vi "Unicode Read Text File Example.vi"() -> ()   [LabVIEW 2020]
doc: "This example demonstrates reading and displaying unicode text from a file."
uses:
  Unicode/Controls/String Encoding.ctl
  Types/UTF-8 Path/UTF-8 Path.lvclass/UTF-8 Path.ctl
  Types/UTF-8 String/UTF-8 String.lvclass/UTF-8 String.ctl
  Types/UTF-8 String/UTF-8 String.lvclass
  Types/UTF-8 Path/UTF-8 Path.lvclass
  815672e0-49fd-43dc-9208-6db65f057bb6.vi
  b6c8d447-eb94-4308-a095-128f48e3c673.vi
  56f3dc87-de23-4d90-98a5-7b236af5e5d4.vi
  45627e68-18eb-4edc-9747-f3175908f235.vi
  Dialog & User Interface/Polymorphic VIs/Write Control Text/Write String Value (UTF-8 String).vi
  Private/Conversion/Text as Encoded Path.vi
  Private/Conversion/Polymorphic VIs/Text as Encoded Path (LabVIEW Path).vi
  Types/UTF-8 Path/Write Encoded UTF-8 Path.vi
  Private/Conversion/Path as Encoded Path.vi
  Private/Conversion/Polymorphic VIs/Path as Encoded Path (LabVIEW Path).vi
  Private/Conversion/String as Encoded String.vi
  Private/Conversion/Polymorphic VIs/String as Encoded String (LabVIEW String).vi
  Private/Conversion/Text as Encoded String.vi
  Private/Conversion/Polymorphic VIs/Text as Encoded String (UTF-8 Path).vi
  Private/Library/gu_open_file_dialog.vi
  Private/Library/gu_select_folder_dialog.vi
  Private/Conversion/Path as UTF-8 Path.vi
  Private/Conversion/Polymorphic VIs/Path as UTF-8 Path (UTF-8 Path).vi
  56f3dc87-de23-4d90-98a5-7b236af5e5d4.vi/8b166e89-7f88-4d33-9f65-0e5b55cfdfba.vi
  56f3dc87-de23-4d90-98a5-7b236af5e5d4.vi/154c5264-acfe-4024-9e59-4207c26e417f.vi
  56f3dc87-de23-4d90-98a5-7b236af5e5d4.vi/a2237eed-bac6-4067-93fc-b5fa504ea8ff.vi
  <vilib>/Utility/error.llb/Clear Errors.vi
  56f3dc87-de23-4d90-98a5-7b236af5e5d4.vi/5e3a38b3-3d0f-4559-ad1c-eed73d89bfdc.vi
  56f3dc87-de23-4d90-98a5-7b236af5e5d4.vi/c6c6a2d4-2ed2-47c1-bb47-bf9afb14d634.vi
  56f3dc87-de23-4d90-98a5-7b236af5e5d4.vi/07ae02c5-2d8e-47e7-881c-96fbd466826f.vi
  56f3dc87-de23-4d90-98a5-7b236af5e5d4.vi/7af25b42-1b06-4de4-a75a-8ed1001daaff.vi
  56f3dc87-de23-4d90-98a5-7b236af5e5d4.vi/e07117c9-d87a-4df6-978c-25aa8b1cd0ee.vi
  File IO/Short Name to Path (Unicode).vi
  Types/UTF-8 Path/New UTF-8 Path.vi
  Unicode/Encode String.vi
  Types/UTF-8 String/Write Encoded UTF-8 String.vi
  Dialog & User Interface/Polymorphic VIs/Write Control Text/Write String Value (UTF-8 String).vi/5206cb6b-04fb-41f5-a37e-29c14f142303.vi
  Private/Conversion/Text to UTF-8.vi
  Private/Conversion/Polymorphic VIs/Text to UTF-8 (LabVIEW Path).vi
  Private/Conversion/Polymorphic VIs/Text to UTF-8 (LabVIEW String).vi
  Types/UTF-8 Path/Read Encoded UTF-8 Path.vi
  Private/Memory/Copy String.vi
  Private/Library/Result To Error.vi
  Private/Conversion/Polymorphic VIs/String as Encoded String (UTF-8 String).vi
  Private/Library/gu_create_file.vi
  56f3dc87-de23-4d90-98a5-7b236af5e5d4.vi/07ae02c5-2d8e-47e7-881c-96fbd466826f.vi/b0de225b-b813-4a3f-91fa-b2c78c384815.vi
  56f3dc87-de23-4d90-98a5-7b236af5e5d4.vi/07ae02c5-2d8e-47e7-881c-96fbd466826f.vi/b1dd94da-e188-4359-85d0-d6693b26af46.vi
  56f3dc87-de23-4d90-98a5-7b236af5e5d4.vi/07ae02c5-2d8e-47e7-881c-96fbd466826f.vi/2799960a-efad-449d-b375-cc5363f1c370.vi
  56f3dc87-de23-4d90-98a5-7b236af5e5d4.vi/07ae02c5-2d8e-47e7-881c-96fbd466826f.vi/2ed7adf8-1da0-426c-b32d-a1b4538e7e16.vi
  Private/Conversion/Text as String.vi
  Private/Conversion/Polymorphic VIs/Text as String (UTF-8 Path).vi
  Private/Library/gu_long_path.vi
  Private/Conversion/Encoded UTF-8 String to Encoded UTF-16LE String.vi
  Unicode/SubVIs/UTF-16 Byte Swap.vi
  Private/Conversion/UTF-8 to Text.vi
  Private/Conversion/Polymorphic VIs/UTF-8 to Text (LabVIEW String).vi
  Private/Conversion/Encoded UTF-16LE String to Encoded UTF-8 String.vi
  Unicode/Prepend BOM.vi
  Private/Conversion/Polymorphic VIs/Text as Encoded String (UTF-8 String).vi
  Private/Memory/Copy String.vi/4d47babd-4a2d-4eb7-b91b-7e707d692665.vi
  Private/Library/gu_free.vi
  Types/UTF-8 String/Read Encoded UTF-8 String.vi
  Unicode/SubVIs/Byte Order Marks.vi
  Unicode/Detect BOM.vi
  <vilib>/Utility/error.llb/Error Cluster From Error Code.vi
  Private/Memory/Copy String Array.vi
  File IO/Path to Short Name (Unicode).vi
  Private/Library/gu_message_box.vi
  Private/User Interface/Write String.vi
  G-Unicode.lvlib
panel:
  out "Raw File Contents":string
  out "Detected Encoding":T1
  out "Encoded File Contents":string
  out "Path":string
  # "Instructions:\n1. Run the VI.\n2. Select a text file which contains unicode text (such as G-Unicode\\Examples\\translation.ini).\n3. The file contents will be read and the encoding detected automatically.\n4. The raw and encoded text contents are displayed."
  # "G"
  # "-Unicode"
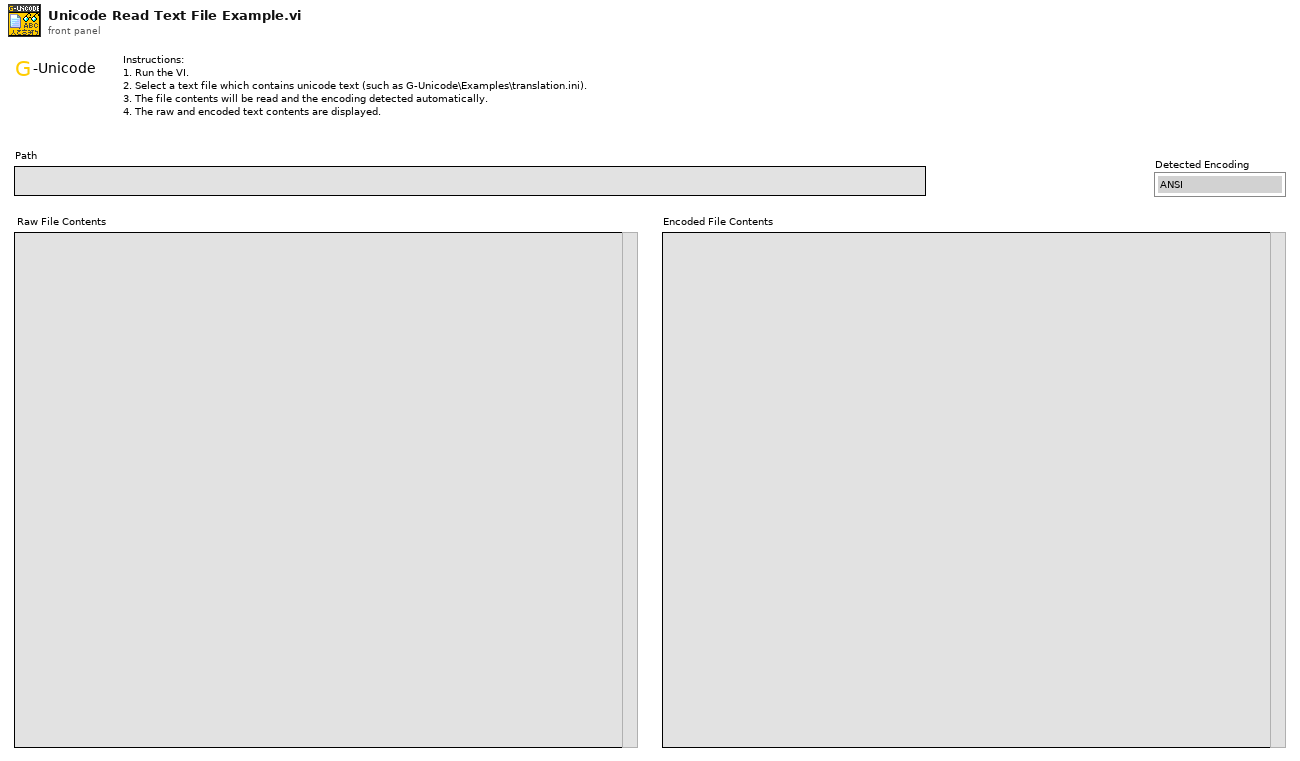
[diagram p1: front panel]
types:
  T1 = typedef "G-Unicode.lvlib/String Encoding.ctl" = enum16{"ANSI", "UTF-8", "UTF-16LE", "UTF-16BE", "Unknown"}
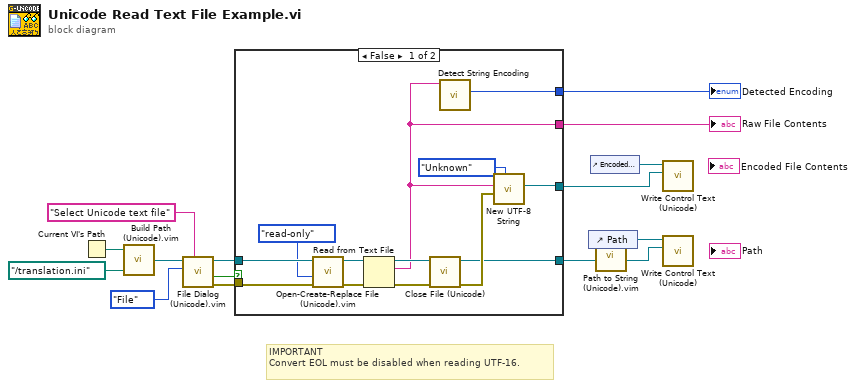
[diagram p0: block diagram]
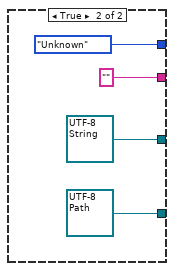
[diagram p2: hidden frame]
diagram:
  # "IMPORTANT\nConvert EOL must be disabled when reading UTF-16."
  n1 = Current VI's Path() -> (path=w3:path)
  n2 = call "Build Path (Unicode).vim"("Base Path"=w3, "Name or Relative Path"=path "../translation.ini") -> ("Appended Path"=w1:refnum<class "UTF-8 Path.lvclass">)  [unwired: 6 in, 1 out]
  n3 = call "File Dialog (Unicode).vim"("Prompt"="Select Unicode text file", "Selection"=enum16{"File", "Multiple Files", "Folder"}."File", "Start Path"=w1) -> ("error out"=w14:errorcluster, "Cancelled"=w13:bool, "Selected Path"=w15:refnum<class "UTF-8 Path.lvclass">)  [unwired: 5 in, 1 out]
  n4 = case shown="False" w13 {
    tunnel: w15 -> [w20 _]
    tunnel: w14 -> [w18 _]
    tunnel: [w24 String_Encoding."Unknown" ("Encoding")] -> w9
    tunnel: [w23 refnum<class "UTF-8 String.lvclass"> refnum ("UTF-8 String")] -> w8
    tunnel: [w22 refnum<class "UTF-8 Path.lvclass"> refnum ("UTF-8 Path")] -> w7
    tunnel: [w21 ""] -> w6
    frame False {
      n5 = call "Open-Create-Replace File (Unicode).vim"("error in"=w18, "Access (0:read/write)"=enum16{"read/write", "read-only", "write-only"}."read-only", "Path (Use Dialog)"=w20) -> ("error out"=w19:errorcluster, "Refnum out"=w17:refnum<file>)  [unwired: 6 in, 1 out]
      n6 = Read from Text File(file (use dialog)=w17, error in=w19) -> (refnum out=w27:refnum<file>, text=w21:string, error out=w26:errorcluster)  [unwired: 2 in, 1 out]
      n7 = call "Close File (Unicode).vi"("error in"=w26, "Refnum"=w27) -> ("error out"=w25:errorcluster, "UTF-8 Path"=w22:refnum<class "UTF-8 Path.lvclass">)  [unwired: 8 in]
      n8 = call "Detect String Encoding.vi"("String"=w21) -> ("Encoding"=w24:T1)  [unwired: 8 in, 2 out]
      n9 = call "New UTF-8 String.vi"("Input Encoding (ANSI)"=String_Encoding."Unknown", "error in"=w25, "String"=w21) -> ("UTF-8 String"=w23:refnum<class "UTF-8 String.lvclass">)  [unwired: 7 in, 1 out]
    }
    frame True {
    }
  }
  "Detected Encoding" <- w9
  "Raw File Contents" <- w6
  n10 = control-ref of="Path"() -> (w11:refnum<vi>)
  n11 = control-ref of="Encoded File Contents"() -> (w10:refnum<vi>)
  n12 = call "Path to String (Unicode).vim"("Path"=w7) -> ("String"=w5:refnum<class "UTF-8 String.lvclass">)  [unwired: 9 in, 1 out]
  n13 = call-poly "Write Control Text (Unicode).vi"("Value"=w8, "Control Ref"=w10) -> ()  [unwired: 9 in, 1 out]
  n14 = call-poly "Write Control Text (Unicode).vi"("Value"=w5, "Control Ref"=w11) -> ()  [unwired: 9 in, 1 out]
